vi "Visa set timeot and termination.vi"(6 "Termination Character Enable":bool, 8 "error in (no error)":errorcluster, 9 "Termination Character":u8, 10 "Timeout Value":u32, 11 "VISA resource name":refnum<visa-resource-name>) -> (0 "error out":errorcluster, 1 "Old Termination Character":u8=13, 2 "Old Timeout Value":u32, 3 "VISA resource name out":refnum<visa-resource-name>, 4 "Old Termination Character Enable":bool)   [LabVIEW 2016]
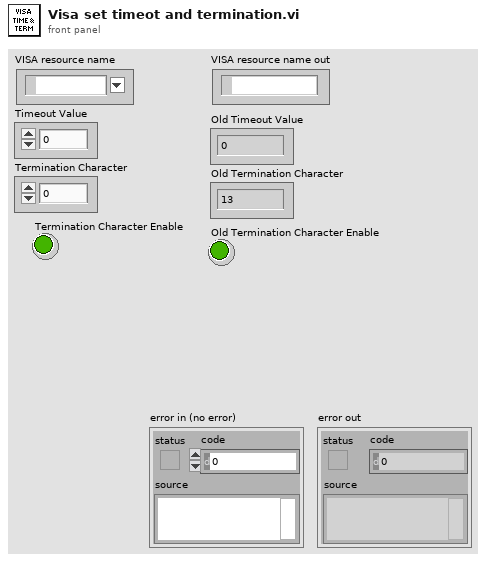
[diagram p1: front panel]
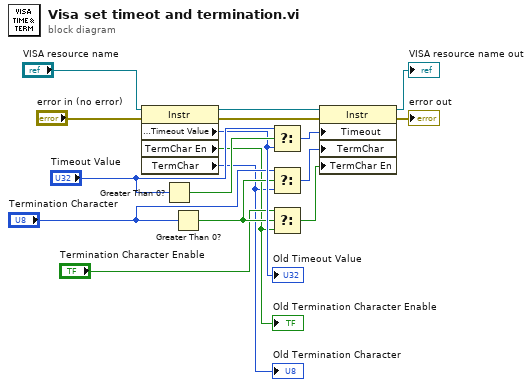
[diagram p0: block diagram]
diagram:
  n1 = property class="Instr"(reference="VISA resource name", error in="error in (no error)") -> (reference out=w16:refnum<visa-resource-name>, error out=w14:errorcluster, "General Settings:Timeout Value"=w9:u32, "TermChar En"=w2:bool, "TermChar"=w1:u8)
  "Old Timeout Value" <- w9
  "Old Termination Character" <- w1
  "Old Termination Character Enable" <- w2
  n2 = Greater Than 0?(x="Timeout Value") -> (x > 0?=w11:bool)
  n3 = Greater Than 0?(x="Termination Character") -> (x > 0?=w5:bool)
  n4 = Select(t="Timeout Value", s=w11, f=w9) -> (s? t:f=w8:u32)
  n5 = Select(t="Termination Character", s=w5, f=w1) -> (s? t:f=w6:u8)
  n6 = Select(t="Termination Character Enable", s=w5, f=w2) -> (s? t:f=w3:bool)
  n7 = property class="Instr"(reference=w16, error in=w14, "Timeout"=w8, "TermChar"=w6, "TermChar En"=w3) -> (reference out=→"VISA resource name out":refnum<visa-resource-name>, error out=→"error out":errorcluster)
